vi "Get Status.vi"(8 "error in (no error)":errorcluster, 11 "DAQmx Base in":refnum<class "NI DAQmx Base.lvclass">) -> (0 "error out":errorcluster, 2 "Status":variant, 3 "DAQmx Base out":refnum<class "NI DAQmx Base.lvclass">)   [LabVIEW 2020, in "NI DAQmx.lvlib" / "NI DAQmx Base.lvclass"]
uses:
  NI DAQmx Base.lvclass
  NI DAQmx Base.lvclass/NI DAQmx Base.ctl
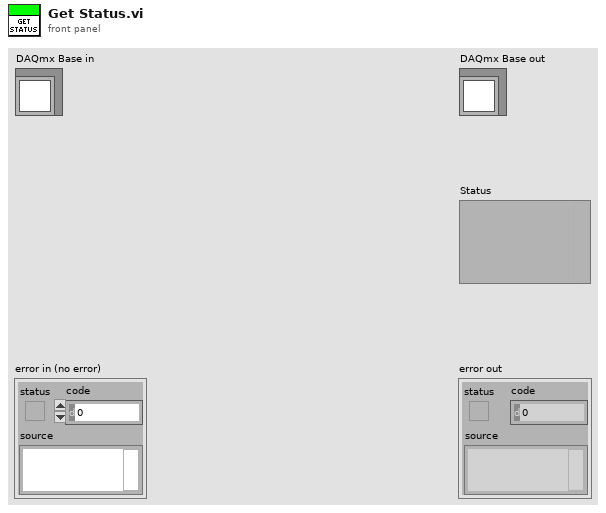
[diagram p1: front panel]
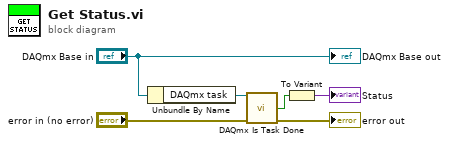
[diagram p0: block diagram]
diagram:
  n1 = Unbundle By Name("DAQmx Base in") -> ("DAQmx task"=w5:refnum<k21>)
  n2 = call <vilib>:"DAQmx Is Task Done.vi"("task/channels in"=w5, "error in"="error in (no error)") -> ("task done?"=w4:bool, "error out"=→"error out":errorcluster)  [unwired: 11 in, 1 out]
  n3 = To Variant(anything=w4) -> (Variant=→"Status":variant)
  "DAQmx Base out" <- "DAQmx Base in"
